vi "Configure channel.vi"(8 "error in (no error)":errorcluster, 10 "Parameters":T1={"Enable Channel (True)"=TRUE, "Channel (0: Channel 1)"=0, "Vertical Coupling (1: DC)"=1, "Probe Attenuation (10: 10X)"=10, "Vertical Range (10.0 V/div)"=10.0, "Vertical Offset (0.0 divs)"=0.0, "Bandwidth (0: MAX Bandwidth)"=0} {"Bandwidth (0: MAX Bandwidth)" items=["MAX Bandwidth", "Unlimited"]; "Probe Attenuation (10: 10X)" items=["1"=1, "10"=10, "20"=20, "50"=50, "100"=100, "500"=500, "1000"=1000]; "Vertical Coupling (1: DC)" items=["AC", "DC", "Ground"]; "Channel (0: Channel 1)" items=["Channel 1", "Channel 2", "Channel 3", "Channel 4", "Math", "Reference A", "Reference B", "Reference C", "Reference D"]}, 11 "Tektonix 2000 in":refnum<class "Tektonix 2000.lvclass">) -> (0 "error out":errorcluster, 3 "Tektonix 2000 out":refnum<class "Tektonix 2000.lvclass">)   [LabVIEW 2020, in "Osciloscope Tektronix.lvlib" / "Tektonix 2000.lvclass"]
uses:
  Tektonix 2000.lvclass
  C:/Users/Pablo/Osciloscope-Tek/TDS2000/Libraries/Osciloscope Tektronix/Clases/Osciloscope/Osciloscope.lvclass
  Osciloscope/Osciloscope.lvclass/Osciloscope.ctl
  Osciloscope/Read COM.vi
  <instrlib>/Tektronix TDS 200 1000 2000 Series/Tektronix TDS 200 1000 2000 Series.lvlib
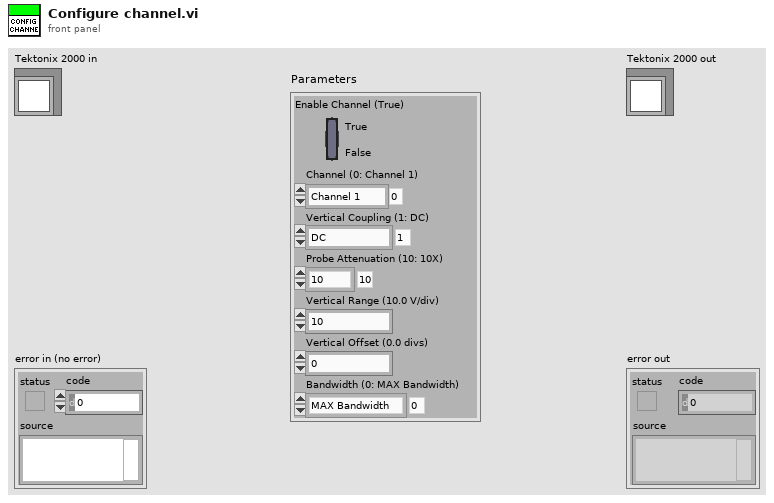
[diagram p1: front panel]
types:
  T1 = cluster{"Enable Channel (True)":bool, "Channel (0: Channel 1)":i32, "Vertical Coupling (1: DC)":i32, "Probe Attenuation (10: 10X)":i32, "Vertical Range (10.0 V/div)":dbl, "Vertical Offset (0.0 divs)":dbl, "Bandwidth (0: MAX Bandwidth)":i32}
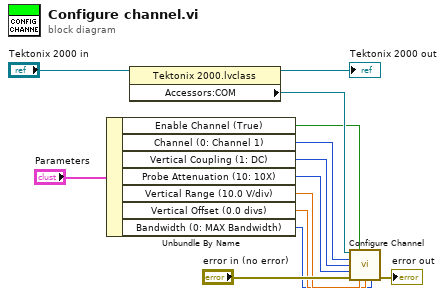
[diagram p0: block diagram]
diagram:
  n1 = Unbundle By Name("Parameters") -> ("Enable Channel (True)"=w7:bool, "Channel (0: Channel 1)"=w6:i32, "Vertical Coupling (1: DC)"=w5:i32, "Probe Attenuation (10: 10X)"=w4:i32, "Vertical Range (10.0 V/div)"=w3:dbl, "Vertical Offset (0.0 divs)"=w2:dbl, "Bandwidth (0: MAX Bandwidth)"=w1:i32)
  n2 = property class="Tektonix 2000.lvclass"(reference="Tektonix 2000 in") -> (reference out=→"Tektonix 2000 out":refnum<class "Tektonix 2000.lvclass">, "Accessors:COM"=w12:refnum<visa-resource-name>)  [unwired: 1 in, 1 out]
  n3 = call <instrlib>:"Configure Channel.vi"("VISA resource name"=w12, "Enable Channel (True)"=w7, "Channel (0: Channel 1)"=w6, "Vertical Coupling (1: DC)"=w5, "Probe Attenuation (10: 10X)"=w4, "error in (no error)"="error in (no error)", "Vertical Range (10.0 V/div)"=w3, "Vertical Offset (0.0 divs)"=w2, "Bandwidth (0: MAX Bandwidth)"=w1) -> ("error out"=→"error out":errorcluster)  [unwired: 5 in, 1 out]
